vi "SMAS_A_LED.vi"() -> ()   [LabVIEW 2018]
uses:
  <vilib>/Platform/TimedLoop/XDataNode/timing_clust.ctl
  <vilib>/Platform/TimedLoop/XDataNode/nitl_modes.ctl
  <vilib>/Platform/TimedLoop/XDataNode/wakeup.ctl
  <vilib>/platform/TimedLoop/XDataNode/XDataNode.xnode
  Program Files (x86)/National Instruments/LabVIEW 2018/examples/Design Patterns/Queued Message Handler/support/QMH Fundamentals - Message Cluster.ctl
  <vilib>/Platform/TimedLoop/XDataNode/XDNodeRunTimeDep.lvlib
  <vilib>/ErrorRing/Error Ring.xnode
  <vilib>/Utility/error.llb/Error Cluster From Error Code.vi
panel:
  out "error out":errorcluster
  in  "stop":bool
  out "SCORE":dbl
  out "HIT!":bool
  in  "SMASH":bool
  out "Display Message":string
  in  "Stop":bool
  in  "Action 2":bool
  in  "Action 1":bool
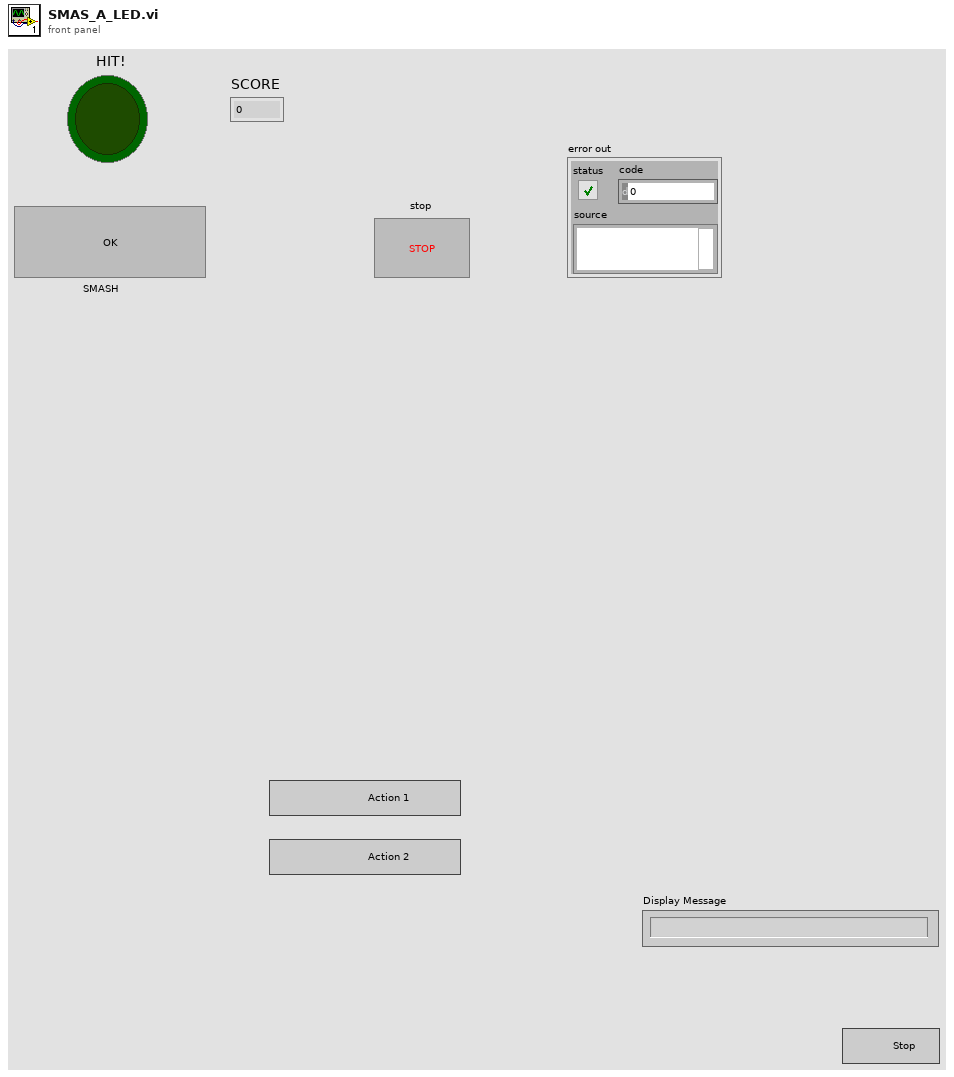
[diagram p1: front panel]
types:
  T1 = typedef "QMH Fundamentals - Message Cluster.ctl" = cluster{"Message":string, "Message Data":variant}
  T2 = typedef "XDNodeRunTimeDep.lvlib/timing_clust.ctl" = cluster{"Expected End [f-1]":u64, "Actual End [f-1]":u64, "Finished Late? [f-1]":bool, "Expected End [i-1]":u64, "Actual End [i-1]":u64, "Finished Late? [i-1]":bool, "Expected Start [i]":u64, "Actual Start [i]":u64, "Expected Start [f]":u64, "Actual Start [f]":u64, "Source Name":string, "Structure Name":string, "Period":i64, "Deadline":i64, "Offset":i64, "Start":i64, "Priority":i32, "Timeout":i32, "Mode":T3, "Wakeup Reason":T4, "Error":errorcluster, "Source Type":string, "Secondary Source Type":string, "Global End Time":u64, "Global Start Time":u64, "Frame Duration":u64, "Iteration Duration":u64, "Assigned CPU":i32, "I/O Scan Engine Mode":u32}
  T3 = typedef "XDNodeRunTimeDep.lvlib/nitl_modes.ctl" = enum32{"No Change", "Process missed periods, maintain original phase", "Discard missed periods, maintain original phase", "Process missed periods, ignore original phase", "Discard missed periods, ignore original phase"}
  T4 = typedef "XDNodeRunTimeDep.lvlib/wakeup.ctl" = enum32{"Normal", "Aborted", "Asynchronous wakeup", "Timing source error", "Timed loop error", "Timeout"}
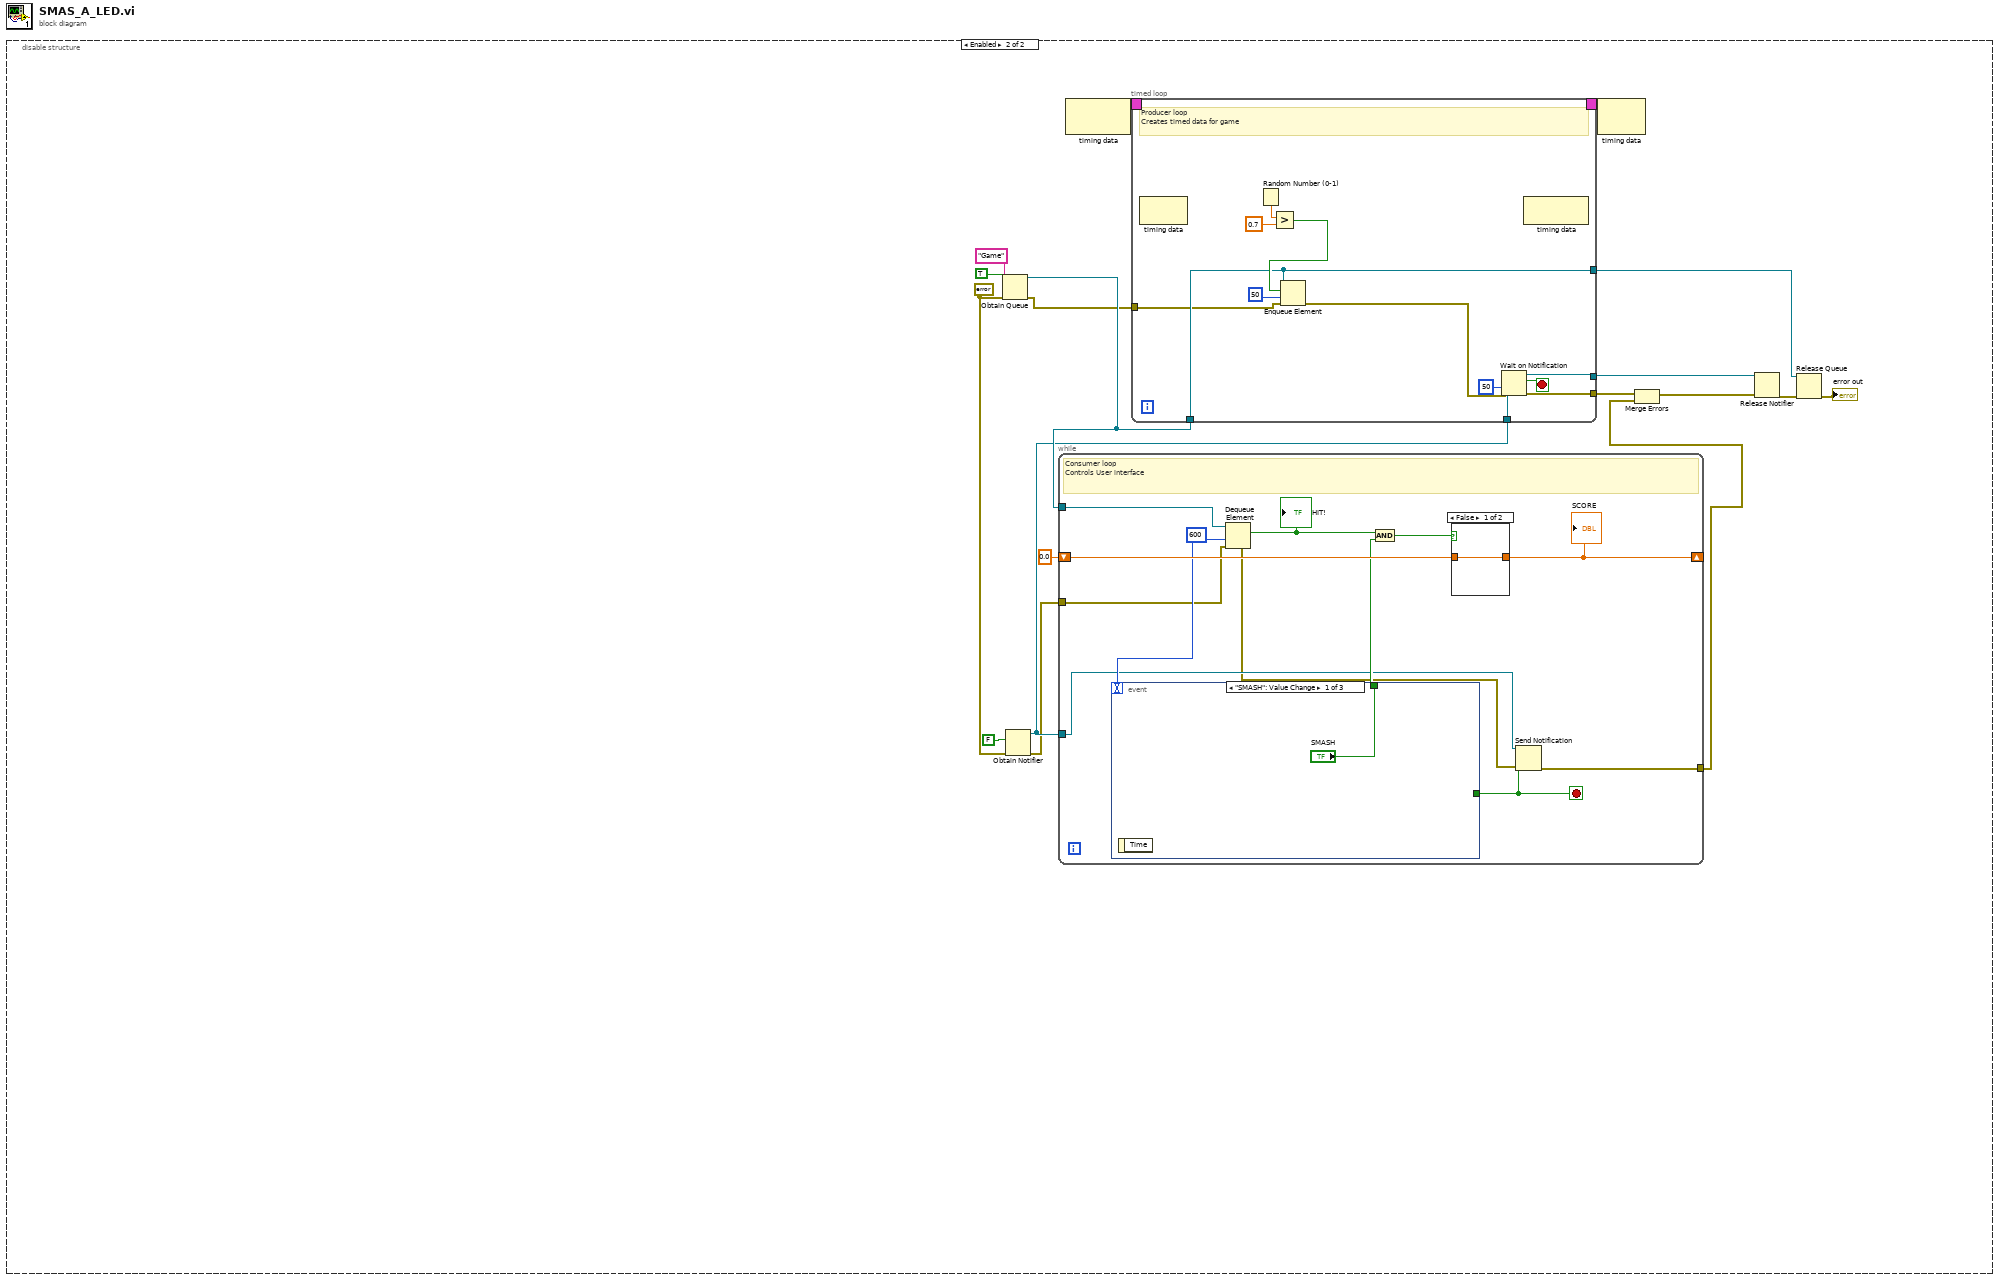
[diagram p0: block diagram]
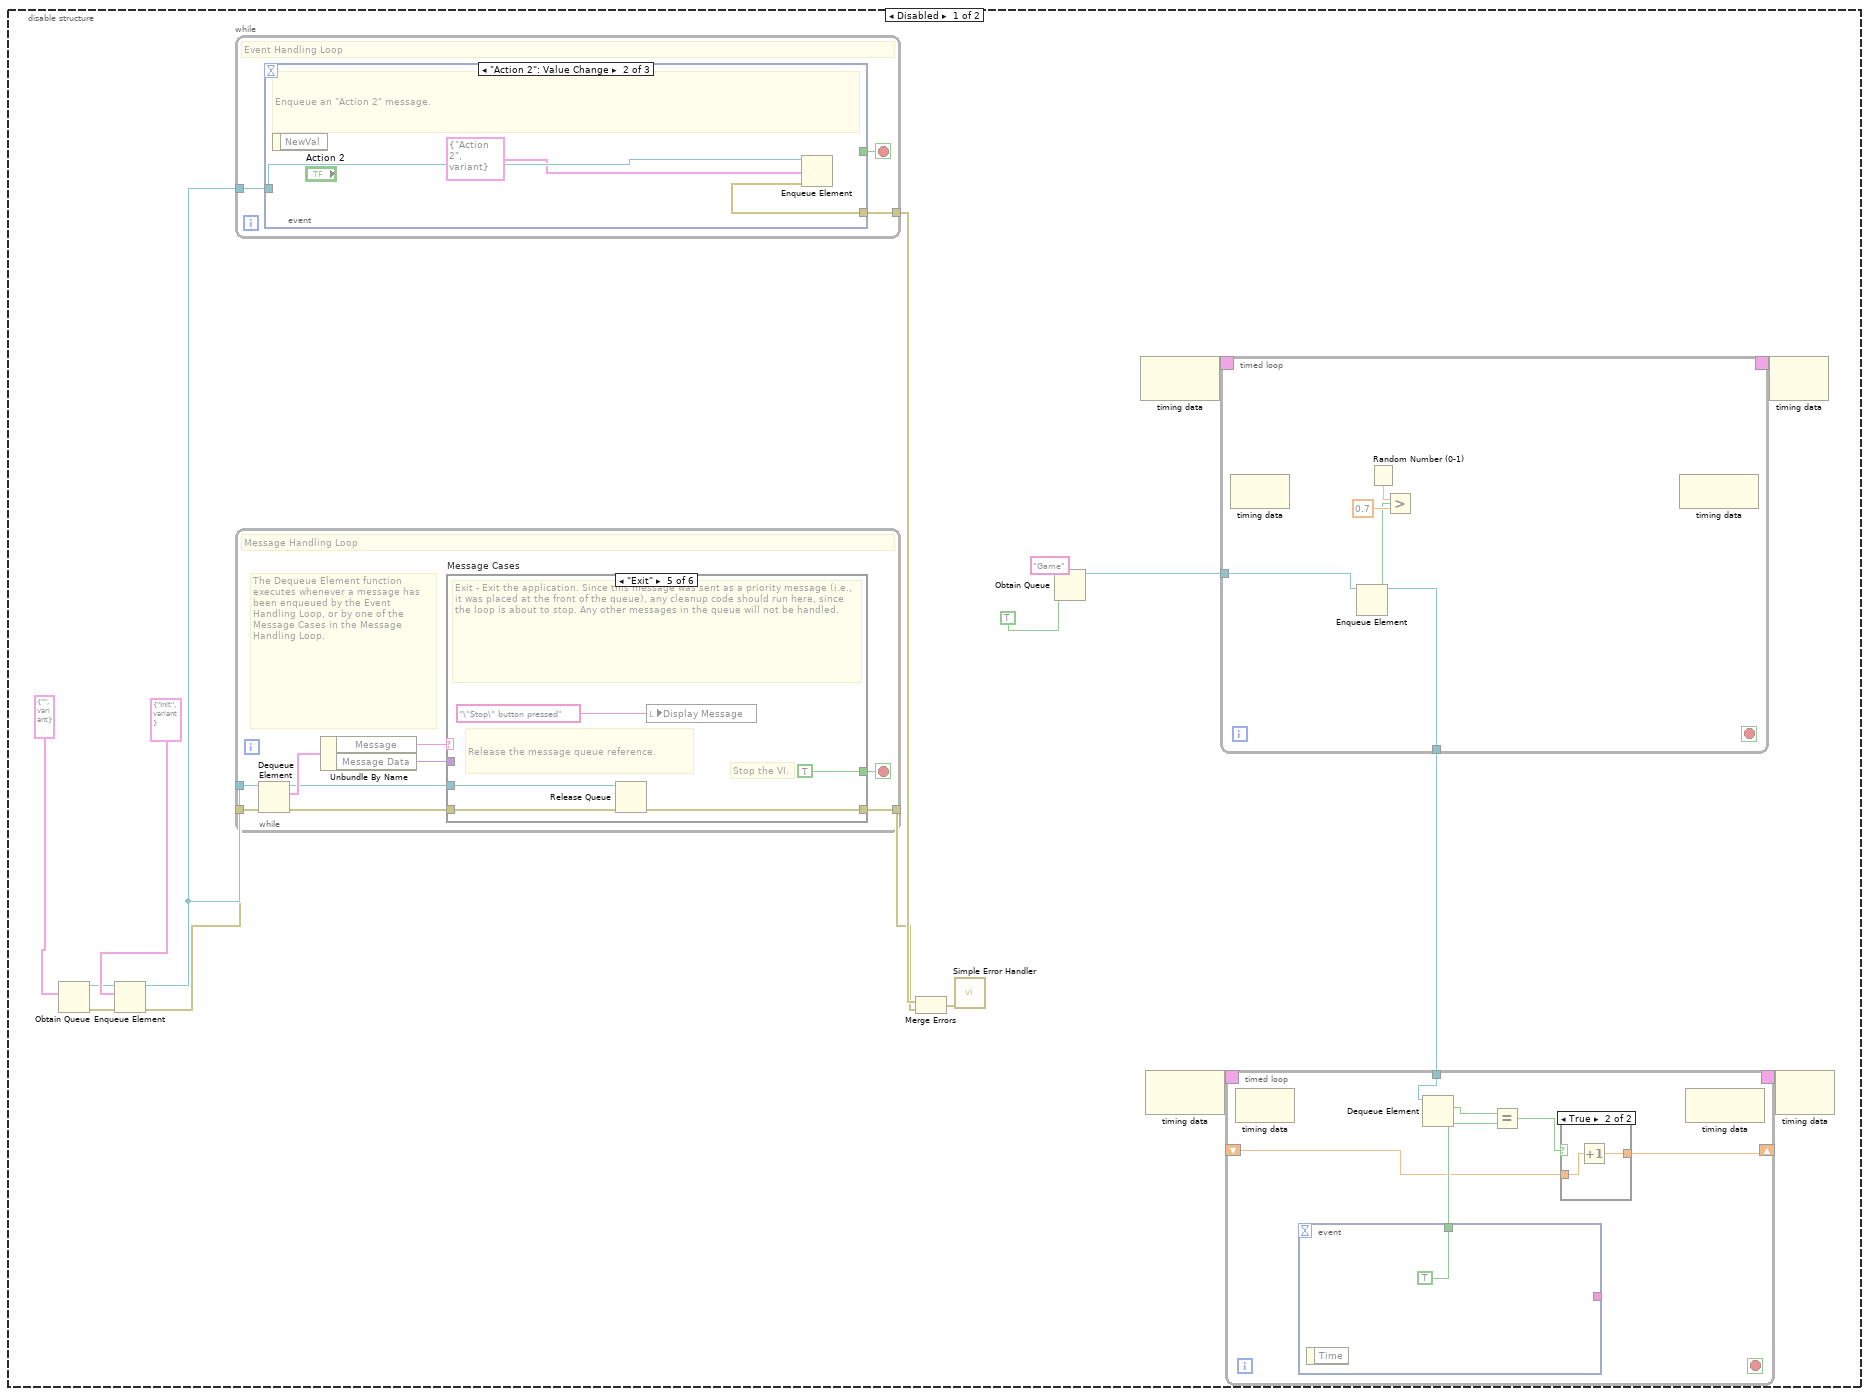
[diagram p2: hidden frame]
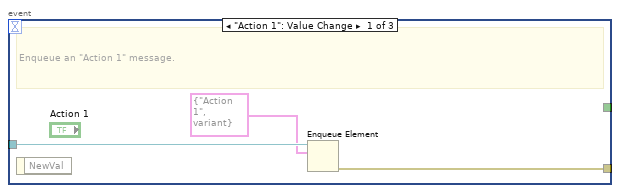
[diagram p4: hidden frame]
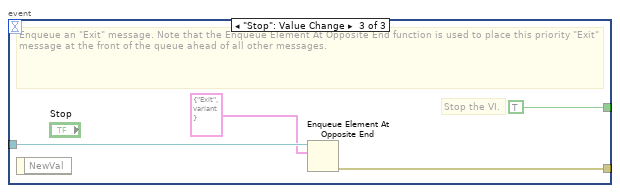
[diagram p5: hidden frame]
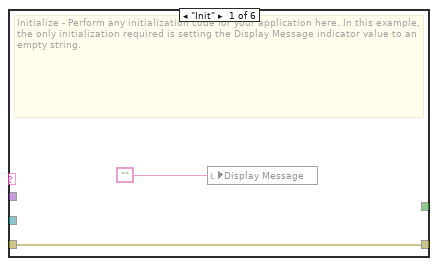
[diagram p6: hidden frame]
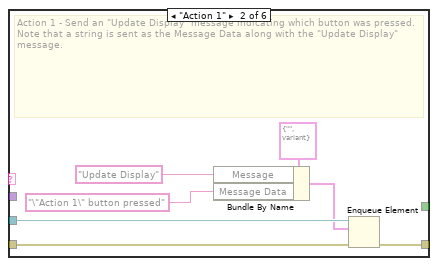
[diagram p7: hidden frame]
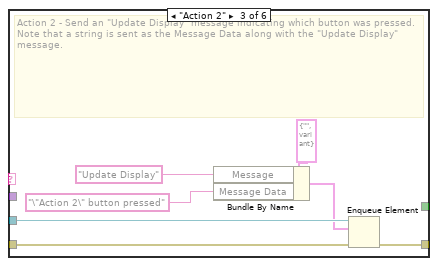
[diagram p8: hidden frame]
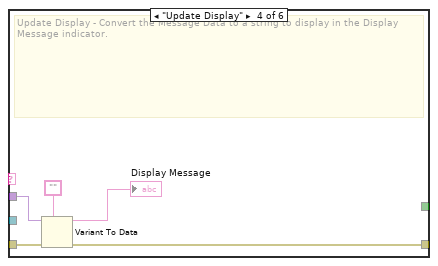
[diagram p9: hidden frame]
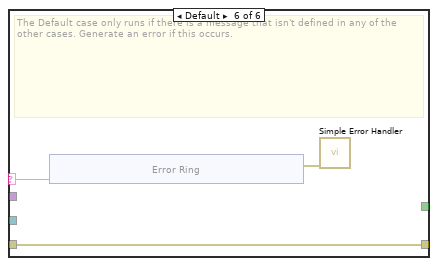
[diagram p10: hidden frame]
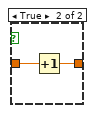
[diagram p11: hidden frame]
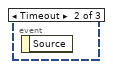
[diagram p12: hidden frame]
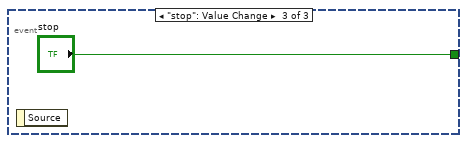
[diagram p13: hidden frame]
diagram:
  n1 = disable-structure shown="Enabled" {
    frame Disabled {
      n2 = Obtain Queue(element data type=T1 {"Message"="", "Message Data"=variant} ("Message Cluster")) -> (queue out=w14:refnum<queue>, error out=w13:errorcluster)  [unwired: 4 in, 1 out]
      n3 = Enqueue Element(queue=w14, element=T1 {"Message"="Init", "Message Data"=variant}, error in (no error)=w13) -> (queue out=w16:refnum<queue>, error out=w15:errorcluster)  [unwired: 1 in, 1 out]
      n4 = while {
        tunnel: w16 -> [w45]
        tunnel: [w43] -> w11
        stop <- w44 stop-if-true
        # "Event Handling Loop"
        n5 = event shown="[1] \"Action 2\": Value Change" {
          selector: _ -> [_ _ _]
          dyn-events: _ -> [_ _ _]
          timeout: _ -> [_ _ _]
          tunnel: [_ _ TRUE] -> w44
          tunnel: w45 -> [w48 w51 w55]
          tunnel: [w47 w50 w54] -> w43
          event "Action 1": Value Change {
            # "Enqueue an \"Action 1\" message."
            n6 = event-data() -> ()  [unwired: 1 in, 1 out]
            n7 = Enqueue Element(queue=w48, element=T1 {"Message"="Action 1", "Message Data"=variant}) -> (error out=w47:errorcluster)  [unwired: 2 in, 2 out]
          }
          event "Action 2": Value Change {
            # "Enqueue an \"Action 2\" message."
            n8 = event-data() -> ()  [unwired: 1 in, 1 out]
            n9 = Enqueue Element(queue=w51, element=T1 {"Message"="Action 2", "Message Data"=variant}) -> (error out=w50:errorcluster)  [unwired: 2 in, 2 out]
          }
          event "Stop": Value Change {
            # "Stop the VI."
            # "Enqueue an \"Exit\" message. Note that the Enqueue Element At Opposite End function is used to place this priority \"Exit\" message at the front of the queue ahead of all other messages."
            n10 = event-data() -> ()  [unwired: 1 in, 1 out]
            n11 = Enqueue Element At Opposite End(queue=w55, element=T1 {"Message"="Exit", "Message Data"=variant}) -> (error out=w54:errorcluster)  [unwired: 2 in, 2 out]
          }
        }
      }
      n12 = while {
        tunnel: w16 -> [w61]
        tunnel: w15 -> [w62]
        tunnel: [w63] -> w10
        stop <- w64 stop-if-true
        # "The Dequeue Element function executes whenever a message has been enqueued by the Event Handling Loop, or by one of the Message Cases in the Message Handling Loop."
        # "Message Handling Loop"
        n13 = Dequeue Element(queue=w61, error in (no error)=w62) -> (queue out=w59:refnum<queue>, element=w60:T1, error out=w58:errorcluster)  [unwired: 1 in, 1 out]
        n14 = Unbundle By Name(w60) -> ("Message"=w57:string, "Message Data"=w56:variant)
        n15 = case "Message Cases" shown="\"Exit\"" w57 {
          selector: w57 -> [_ _ _ _ _ w93]
          tunnel: w59 -> [_ w73 w80 _ w90 _]
          tunnel: w58 -> [w66 w71 w78 w85 w87 w92]
          tunnel: [w66 w72 w79 w82 w88 w92] -> w63
          tunnel: [_ _ _ _ TRUE _] -> w64
          tunnel: w56 -> [_ _ _ w84 _ _]
          frame "Init" {
            # "Initialize - Perform any initialization code for your application here. In this example, the only initialization required is setting the Display Message indicator value to an empty string."
            n16 = local write "Display Message"("") -> ()
          }
          frame "Action 1" {
            # "Action 1 - Send an \"Update Display\" message indicating which button was pressed. Note that a string is sent as the Message Data along with the \"Update Display\" message."
            n17 = Bundle By Name(cluster=T1 {"Message"="", "Message Data"=variant} ("Message Cluster"), "Message"="Update Display", "Message Data"="\"Action 1\" button pressed" ("L10n_Action 1 Pressed")) -> (w68:T1)
            n18 = Enqueue Element(queue=w73, element=w68, error in (no error)=w71) -> (error out=w72:errorcluster)  [unwired: 1 in, 2 out]
          }
          frame "Action 2" {
            # "Action 2 - Send an \"Update Display\" message indicating which button was pressed. Note that a string is sent as the Message Data along with the \"Update Display\" message."
            n19 = Bundle By Name(cluster=T1 {"Message"="", "Message Data"=variant} ("Message Cluster"), "Message"="Update Display", "Message Data"="\"Action 2\" button pressed" ("L10n_Action 2 Pressed")) -> (w75:T1)
            n20 = Enqueue Element(queue=w80, element=w75, error in (no error)=w78) -> (error out=w79:errorcluster)  [unwired: 1 in, 2 out]
          }
          frame "Update Display" {
            # "Update Display - Convert the Message Data to a string to display in the Display Message indicator."
            n21 = Variant To Data(error in=w85, type="", Variant=w84) -> (data=→"Display Message":string, error out=w82:errorcluster)
          }
          frame "Exit" {
            # "Stop the VI."
            # "Release the message queue reference."
            # "Exit - Exit the application. Since this message was sent as a priority message (i.e., it was placed at the front of the queue), any cleanup code should run here, since the loop is about to stop. Any other messages in the queue will not be handled."
            n22 = Release Queue(queue=w90, error in (no error)=w87) -> (error out=w88:errorcluster)  [unwired: 1 in, 2 out]
            n23 = local write "Display Message"("\"Stop\" button pressed" ("L10n_Stop Pressed")) -> ()
          }
          frame Default {
            # "The Default case only runs if there is a message that isn't defined in any of the other cases. Generate an error if this occurs."
            n24 = xnode "Error Ring"("parameter 0"=w93) -> ("error out"=w91:errorcluster)
            n25 = call <vilib>:"Simple Error Handler.vi"("error in (no error)"=w91) -> ()  [unwired: 4 in, 5 out]
          }
        }
      }
      n26 = Merge Errors(w11, w10) -> (w18:errorcluster)
      n27 = call <vilib>:"Simple Error Handler.vi"("error in (no error)"=w18) -> ()  [unwired: 4 in, 5 out]
      n28 = Obtain Queue(name (unnamed)="Game", element data type=TRUE) -> (queue out=w3:refnum<queue>)  [unwired: 3 in, 2 out]
      n29 = node-c288() -> (w9:T2)  [unwired: 1 in]
      n30 = node-c288() -> (w7:T2)  [unwired: 1 in]
      n31 = timed-loop {
        timing: w9 -> [_]
        timing-out: [_] -> w8
        tunnel: w3 -> [w36]
        tunnel: [w34] -> w2
        stop <- _ stop-if-true
        n32 = node-c288() -> ()  [unwired: 1 in, 1 out]
        n33 = Random Number (0-1)() -> (number: 0 to 1=w38:dbl)
        n34 = Greater?(x=w38, y=0.7) -> (0:w35:bool)
        n35 = Enqueue Element(queue=w36, element=w35) -> (queue out=w34:refnum<queue>)  [unwired: 2 in, 2 out]
        n36 = node-c288() -> ()  [unwired: 1 in, 1 out]
      }
      n37 = timed-loop {
        timing: w7 -> [_]
        timing-out: [_] -> w6
        tunnel: w2 -> [w24]
        shift-right: [w21] -> w1
        shift-left: _ -> [w20]
        stop <- _ stop-if-true
        n38 = node-c288() -> ()  [unwired: 1 in, 1 out]
        n39 = event {
          selector: _ -> [_]
          dyn-events: _ -> [_]
          timeout: _ -> [_]
          tunnel: [_] -> w25
          tunnel: [TRUE] -> w22
          event #0 {
            n40 = event-data() -> ()  [unwired: 1 in, 1 out]
          }
        }
        n41 = Dequeue Element(queue=w24) -> (element=w23:bool)  [unwired: 2 in, 3 out]
        n42 = Equal?(x=w23, y=w22) -> (x = y?=w19:bool)
        n43 = case shown="True" w19 {
          tunnel: [w26 w28] -> w21
          tunnel: w20 -> [w26 w27]
          frame False {
          }
          frame True {
            n44 = Increment(x=w27) -> (x+1=w28:dbl)
          }
        }
        n45 = node-c288() -> ()  [unwired: 1 in, 1 out]
      }
      n46 = node-c288(w8) -> ()  [unwired: 1 out]
      n47 = node-c288(w6) -> ()  [unwired: 1 out]
    }
    frame Enabled {
      w104 = errorcluster {"status"=FALSE, "code"=0, "source"=""} ("error in (no error)")
      n48 = Obtain Queue(name (unnamed)="Game", element data type=TRUE, error in (no error)=w104) -> (queue out=w113:refnum<queue>, error out=w101:errorcluster)  [unwired: 2 in, 1 out]
      n49 = Obtain Notifier(notification data type=FALSE, error in (no error)=w104) -> (notifier out=w110:refnum<notifier>, error out=w103:errorcluster)  [unwired: 2 in, 1 out]
      n50 = while {
        shift-right: [w125] -> _
        shift-left: 0.0 -> [w128]
        tunnel: w113 -> [w126]
        tunnel: w110 -> [w122]
        tunnel: [w121] -> w102
        tunnel: w103 -> [w120]
        stop <- w123 stop-if-true
        w124 = 600 ("timeout in ms (-1)")
        # "Consumer loop\nControls User interface"
        n51 = event shown="[0] \"SMASH\": Value Change" {
          selector: _ -> [_ _ _]
          dyn-events: _ -> [_ _ _]
          timeout: w124 -> [_ _ _]
          tunnel: ["SMASH" _ _] -> w127
          tunnel: [_ _ "stop"] -> w123
          event "SMASH": Value Change {
            n52 = event-data() -> ()  [unwired: 1 in, 1 out]
          }
          event Timeout {
            n53 = event-data() -> ()  [unwired: 1 in, 1 out]
          }
          event "stop": Value Change {
            n54 = event-data() -> ()  [unwired: 1 in, 1 out]
          }
        }
        n55 = Dequeue Element(queue=w126, timeout in ms (-1)=w124, error in (no error)=w120) -> (element=w130:bool, error out=w119:errorcluster)  [unwired: 2 out]
        "HIT!" <- w130
        n56 = And(x=w130, y=w127) -> (x .and. y?=w129:bool)
        n57 = case shown="False" w129 {
          tunnel: [w131 w133] -> w125
          tunnel: w128 -> [w131 w132]
          frame False {
          }
          frame True {
            n58 = Increment(x=w132) -> (x+1=w133:dbl)
          }
        }
        "SCORE" <- w125
        n59 = Send Notification(notification=w123, notifier=w122, error in (no error)=w119) -> (error out=w121:errorcluster)  [unwired: 1 out]
      }
      n60 = node-c288() -> (w118:T2)  [unwired: 1 in]
      n61 = timed-loop {
        timing: w118 -> [_]
        timing-out: [_] -> w117
        tunnel: w113 -> [w138]
        tunnel: [w142] -> w111
        tunnel: w110 -> [w140]
        tunnel: [w139] -> w109
        tunnel: [w138] -> w106
        tunnel: w101 -> [w137]
        stop <- w143 stop-if-true
        # "Producer loop \nCreates timed data for game"
        n62 = node-c288() -> ()  [unwired: 1 in, 1 out]
        n63 = Random Number (0-1)() -> (number: 0 to 1=w147:dbl)
        n64 = Greater?(x=w147, y=0.7) -> (0:w145:bool)
        n65 = Enqueue Element(queue=w138, element=w145, timeout in ms (-1)=50, error in (no error)=w137) -> (error out=w136:errorcluster)  [unwired: 2 out]
        n66 = Wait on Notification(notifier=w140, timeout in ms (-1)=50, error in (no error)=w136) -> (notifier out=w142:refnum<notifier>, notification=w143:bool, error out=w139:errorcluster)  [unwired: 1 in, 1 out]
        n67 = node-c288() -> ()  [unwired: 1 in, 1 out]
      }
      n68 = node-c288(w117) -> ()  [unwired: 1 out]
      n69 = Merge Errors(w109, w102) -> (w108:errorcluster)
      n70 = Release Notifier(notifier=w111, error in (no error)=w108) -> (error out=w107:errorcluster)  [unwired: 1 in, 2 out]
      n71 = Release Queue(queue=w106, error in (no error)=w107) -> (error out=→"error out":errorcluster)  [unwired: 1 in, 2 out]
    }
  }
